vi "text width.vi"(11 "text":string) -> (3 "Min Cell Width":u32)   [LabVIEW 2021, in "RocketPlot.lvlib" / "TipTablePanel.lvclass"]
uses:
  TipTablePanel.lvclass
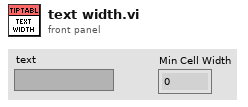
[diagram p1: front panel]
types:
  T1 = cluster{"Font Name:":string, "Size":i16, "Strikeout?":bool, "Italic?":bool, "Underline?":bool, "Outline?":bool, "Shadow?":bool, "Bold?":bool}
  T2 = enum16{"User-specified Font", "Application Font", "System Font", "Dialog Font"}
  T3 = cluster{"left":i16, "top":i16, "right":i16, "bottom":i16}
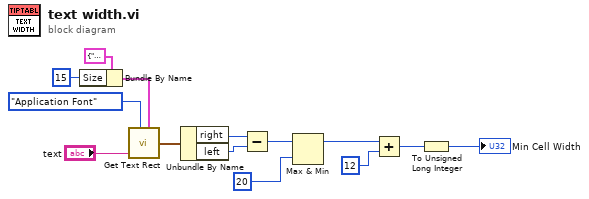
[diagram p0: block diagram]
diagram:
  n1 = Bundle By Name(cluster=T1 {"Font Name:"="", "Size"=0, "Strikeout?"=FALSE, "Italic?"=FALSE, "Underline?"=FALSE, "Outline?"=FALSE, "Shadow?"=FALSE, "Bold?"=FALSE} ("[user-specified font]"), "Size"=i16 15) -> (w9:T1)
  n2 = call <vilib>:"Get Text Rect.vi"("desired font(Application)"=T2."Application Font", "text"="text", "[user-specified font]"=w9) -> ("rect"=w6:T3)  [unwired: 6 in]
  n3 = Unbundle By Name(w6) -> ("right"=w7:i16, "left"=w8:i16)
  n4 = Subtract(x=w7, y=w8) -> (x-y=w5:i16)
  n5 = Max & Min(x=w5, y=i16 20) -> (max(x,y)=w3:i16)  [unwired: 1 out]
  n6 = Add(x=w3, y=i16 12) -> (x+y=w13:i16)
  n7 = To Unsigned Long Integer(number=w13) -> (unsigned 32bit integer=→"Min Cell Width":u32)
